vi "average demodulated.vi"(4 "Demodulated signal":dbl[][](array[numeric])) -> (1 "Demodulated averaged":dbl[](array[numeric]))   [LabVIEW 2011]
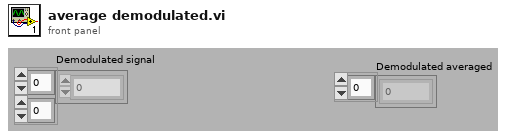
[diagram p1: front panel]
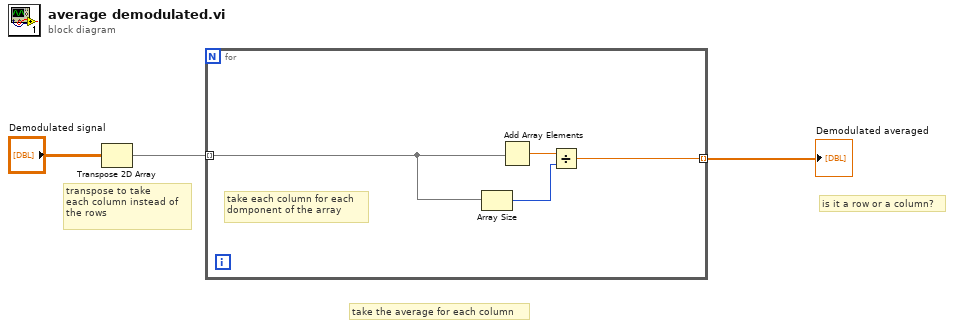
[diagram p0: block diagram]
diagram:
  # "is it a row or a column?"
  # "transpose to take \neach column instead of\nthe rows"
  # "take the average for each column"
  n1 = Transpose 2D Array(2D array="Demodulated signal") -> (transposed array=w1:dbl[][])
  n2 = for {
    tunnel: [w7] -> w3 mode=indexing
    tunnel: w1 -> [w4] mode=indexing
    # "take each column for each\ndomponent of the array"
    n3 = Array Size(array=w4) -> (size(s)=w5:i32)
    n4 = Add Array Elements(numeric array=w4) -> (sum=w6:dbl)
    n5 = Divide(x=w6, y=w5) -> (x/y=w7:dbl)
  }
  "Demodulated averaged" <- w3
